vi "Pachube PUT EEML Format LaunchPad-v2.vi"(7 "tag":string="0", 8 "max_value":dbl, 9 "min_value":dbl, 10 "data id":string="0", 11 "current_value":dbl) -> (1 "Data":string)   [LabVIEW 2011]
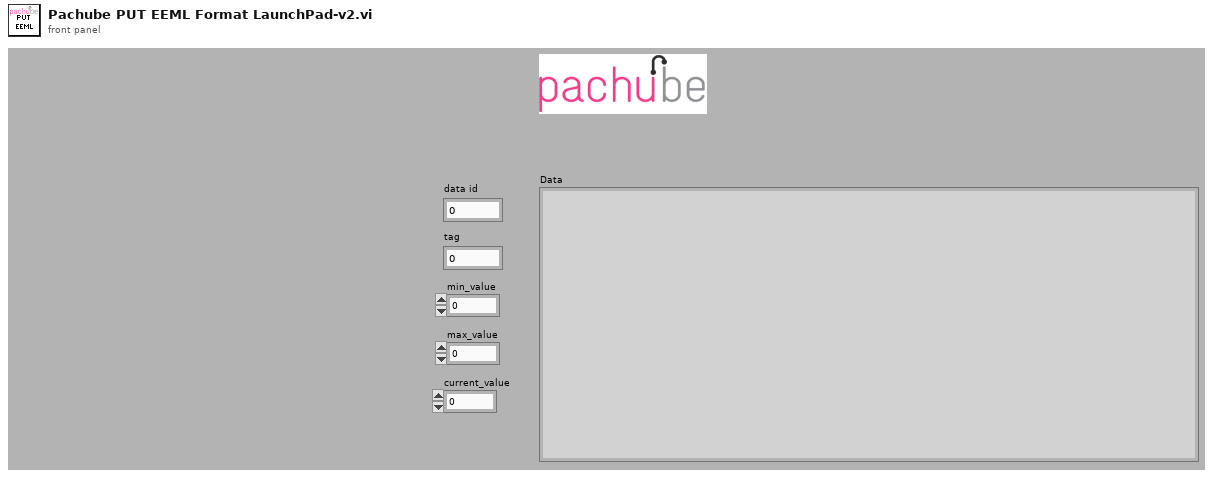
[diagram p1: front panel]
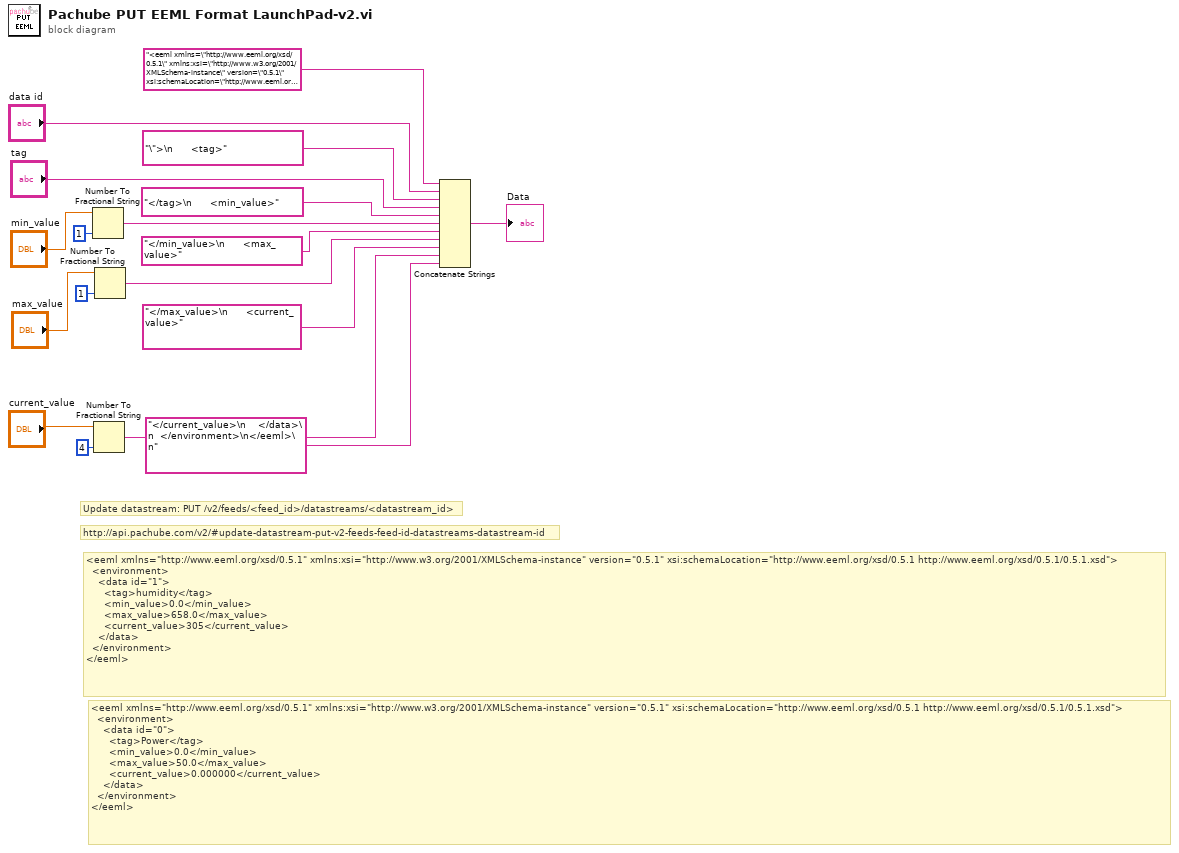
[diagram p0: block diagram]
diagram:
  # "<eeml xmlns=\"http://www.eeml.org/xsd/0.5.1\" xmlns:xsi=\"http://www.w3.org/2001/XMLSchema-instance\" version=\"0.5.1\" xsi:schemaLocation=\"http://www.eeml.org/xsd/0.5.1 http://www.eeml.org/xsd/0.5.1/0.5.1.xsd\">\n  <environment>\n    <data id=\"0\">\n      <tag>Power</tag>\n      <min_value>0.0</min_value>\n      <max_value>50.0</max_value>\n      <current_value>0.000000</current_value>\n    </data>\n  </environment>\n</eeml>"
  # "Update datastream: PUT /v2/feeds/<feed_id>/datastreams/<datastream_id>"
  # "http://api.pachube.com/v2/#update-datastream-put-v2-feeds-feed-id-datastreams-datastream-id"
  # "<eeml xmlns=\"http://www.eeml.org/xsd/0.5.1\" xmlns:xsi=\"http://www.w3.org/2001/XMLSchema-instance\" version=\"0.5.1\" xsi:schemaLocation=\"http://www.eeml.org/xsd/0.5.1 http://www.eeml.org/xsd/0.5.1/0.5.1.xsd\">\n  <environment>\n    <data id=\"1\">\n      <tag>humidity</tag>\n      <min_value>0.0</min_value>\n      <max_value>658.0</max_value>\n      <current_value>305</current_value>\n    </data>\n  </environment>\n</eeml>"
  n1 = Number To Fractional String(number="min_value", precision (6)=i16 1) -> (F-format string=w7:string)  [unwired: 2 in]
  n2 = Number To Fractional String(number="current_value", precision (6)=i16 4) -> (F-format string=w15:string)  [unwired: 2 in]
  n3 = Number To Fractional String(number="max_value", precision (6)=i16 1) -> (F-format string=w4:string)  [unwired: 2 in]
  n4 = Concatenate Strings("<eeml xmlns=\"http://www.eeml.org/xsd/0.5.1\" xmlns:xsi=\"http://www.w3.org/2001/XMLSchema-instance\" version=\"0.5.1\" xsi:schemaLocation=\"http://www.eeml.org/xsd/0.5.1 http://www.eeml.org/xsd/0.5.1/0.5.1.xsd\">\n  <environment>\n    <data id=\"", "data id", "\">\n      <tag>", "tag", "</tag>\n      <min_value>", w7, "</min_value>\n      <max_value>", w4, "</max_value>\n      <current_value>", w15, "</current_value>\n    </data>\n  </environment>\n</eeml>\n") -> (→"Data":string)
